vi "RPC Download Component.vi"(8 "error in (no error)":errorcluster, 10 "Component Path (empty)":path, 11 "Client (\"\")":string) -> (0 "error out":errorcluster)   [LabVIEW 2011]
uses:
  OpenG/file/file.llb/File Exists - Scalar__ogtk.vi
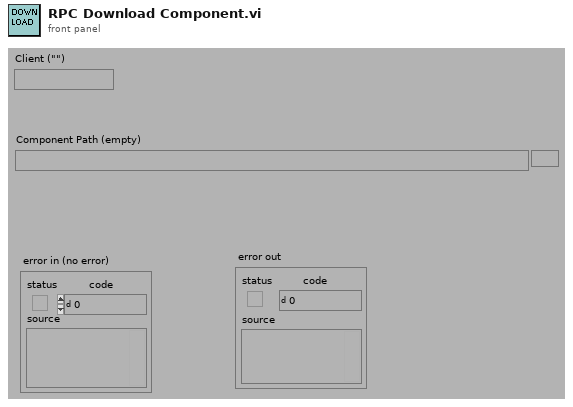
[diagram p1: front panel]
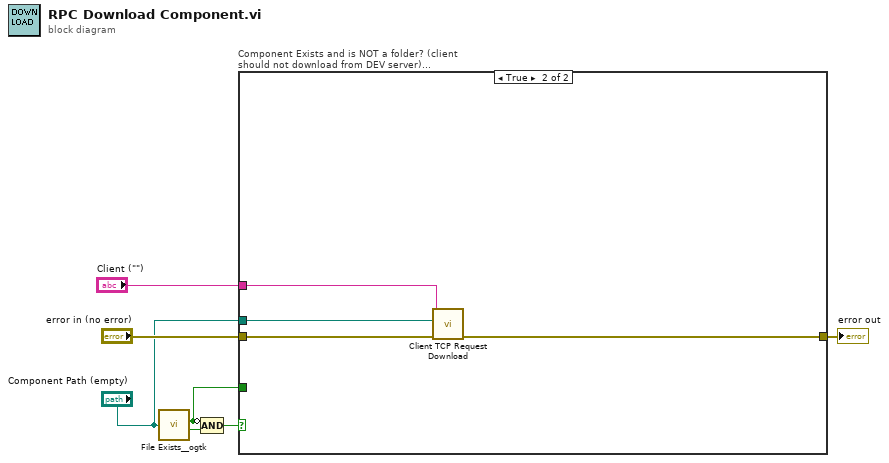
[diagram p0: block diagram]
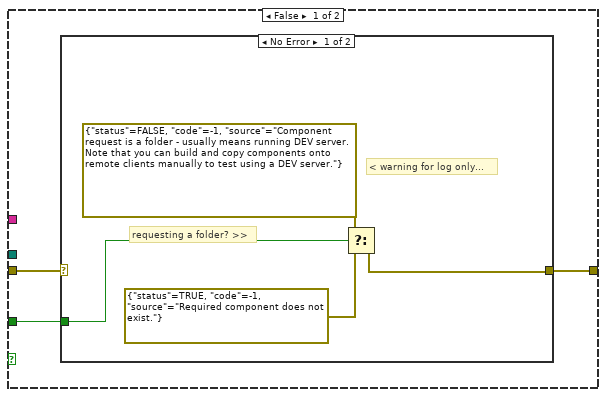
[diagram p2: hidden frame]
diagram:
  n1 = call-poly "File Exists__ogtk.vi"("file path"="Component Path (empty)") -> ("is directory"=w2:bool, "exists"=w6:bool)  [unwired: 6 in]
  n2 = Compound Arithmetic op=AND(invert w2, w6) -> (w4:bool)
  n3 = case "Component Exists and is NOT a folder? (client should not download from DEV server)..." shown="True" w4 {
    tunnel: [w9 w18] -> w7
    tunnel: "Component Path (empty)" -> [_ w17]
    tunnel: "error in (no error)" -> [w10 w19]
    tunnel: "Client (\"\")" -> [_ w16]
    tunnel: w2 -> [w8 _]
    frame False {
      n4 = case shown="No Error" w10 {
        selector: w10 -> [_ w15]
        tunnel: [w12 w15] -> w9
        tunnel: w8 -> [w14 _]
        frame No Error {
          # "< warning for log only..."
          # "requesting a folder? >>"
          n5 = Select(t=errorcluster {"status"=FALSE, "code"=-1, "source"="Component request is a folder - usually means running DEV server.  Note that you can build and copy components onto remote clients manually to test using a DEV server."} ("error IO"), s=w14, f=errorcluster {"status"=TRUE, "code"=-1, "source"="Required component does not exist."} ("error IO")) -> (s? t:f=w12:errorcluster)
        }
        frame Error {
        }
      }
    }
    frame True {
      n6 = call "Client TCP Request Download.vi"("error in (no error)"=w19, "File URL (empty)"=w17, "Client (\"\": localhost)"=w16) -> ("error out"=w18:errorcluster)  [unwired: 8 out]
    }
  }
  "error out" <- w7
